vi "Read Voltage Number Select.vi"(8 "error in (no error)":errorcluster, 11 "Generic Power Analyzer in":refnum<class "Generic Power Analyzer.lvclass">) -> (0 "error out":errorcluster, 2 "Voltage Number Select":u16, 3 "Generic Power Analyzer out":refnum<class "Generic Power Analyzer.lvclass">)   [LabVIEW 2016, in "Generic Power Analyzer.lvlib" / "Generic Power Analyzer.lvclass"]
uses:
  Generic Power Analyzer.lvclass
  Generic Power Analyzer.lvclass/Generic Power Analyzer.ctl
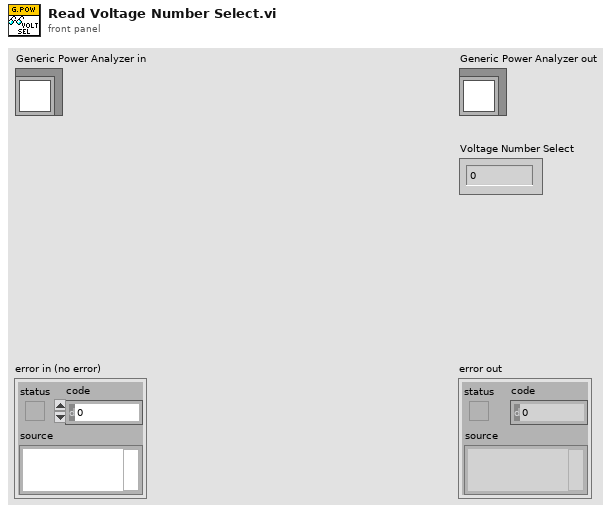
[diagram p1: front panel]
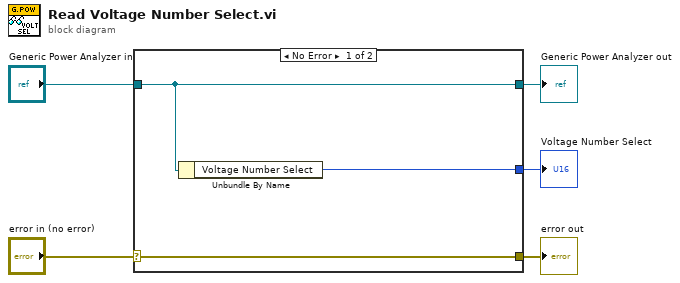
[diagram p0: block diagram]
diagram:
  n1 = case shown="No Error" "error in (no error)" {
    selector: "error in (no error)" -> [w8 w9]
    tunnel: [w8 w9] -> w4
    tunnel: [w7 w10] -> w2
    tunnel: "Generic Power Analyzer in" -> [w7 w10]
    tunnel: [w6 _] -> w1
    frame No Error {
      n2 = Unbundle By Name(w7) -> ("Voltage Number Select"=w6:u16)
    }
    frame Error {
    }
  }
  "error out" <- w4
  "Generic Power Analyzer out" <- w2
  "Voltage Number Select" <- w1
